vi "ReadData_9234.vi"(8 "error in":errorcluster, 11 "Module Config Selector":i16) -> (0 "error out":errorcluster, 3 "Data Array":sgl[](array[numeric]) format="%.2f")   [LabVIEW 2017, in "BOP_VibAPI_4.lvlib"]
uses:
  <vilib>/addons/InsightCM/Devices/Shared/Cms/Fpga/Acquisition/source/subVIs/VibAPI_4/BOP_VibAPI_4.lvlib
  <vilib>/rvi/eio/common/nirviEmuTemplateMethod_errors.vi
  <vilib>/eio/EIONode/EIONode.xnode
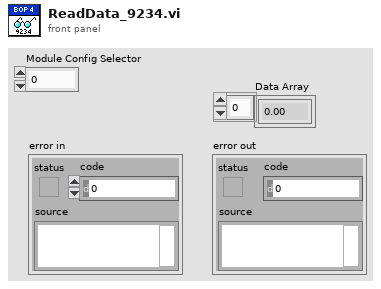
[diagram p1: front panel]
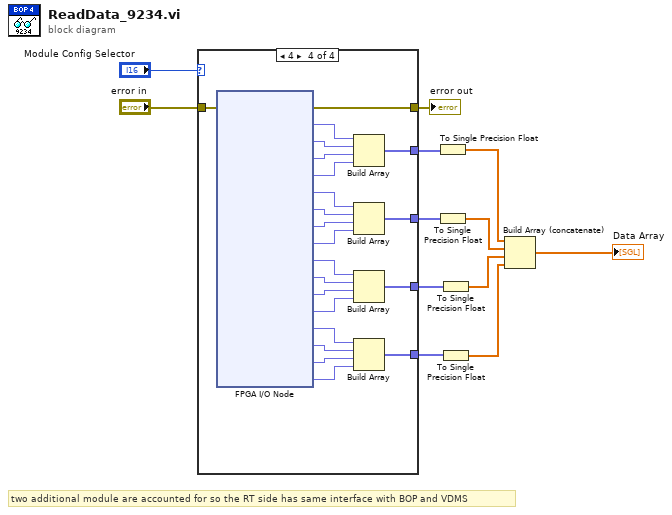
[diagram p0: block diagram]
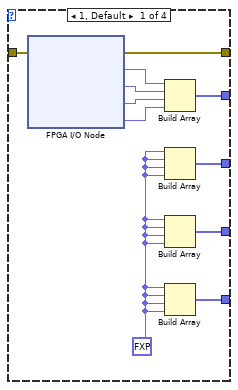
[diagram p2: hidden frame]
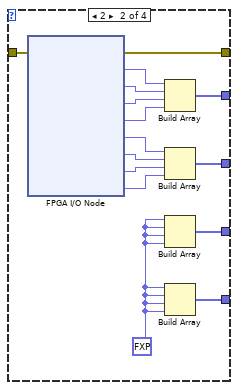
[diagram p3: hidden frame]
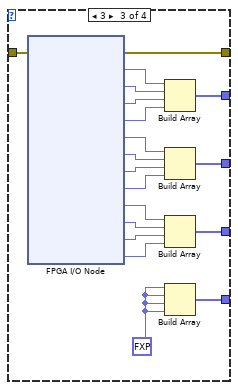
[diagram p4: hidden frame]
diagram:
  # "two additional module are accounted for so the RT side has same interface with BOP and VDMS"
  n1 = case shown="4" "Module Config Selector" {
    tunnel: "error in" -> [w20 w35 w54 w76]
    tunnel: [w19 w34 w53 w75] -> w11
    tunnel: [w18 w33 w52 w74] -> w8
    tunnel: [w17 w32 w51 w73] -> w6
    tunnel: [w16 w31 w50 w72] -> w4
    tunnel: [w15 w27 w43 w62] -> w2
    frame 1, Default {
      w13 = fxp<+/-,24,7> 0.0 ("Mod3/AI2")
      n2 = xnode "FPGA I/O Node"("error in"=w20) -> ("error out"=w19:errorcluster, "Mod1/AI0"=w21:fxp<+/-,24,4>, "Mod1/AI1"=w23:fxp<+/-,24,4>, "Mod1/AI2"=w22:fxp<+/-,24,4>, "Mod1/AI3"=w14:fxp<+/-,24,4>)  [unwired: 4 in, 4 out]
      n3 = Build Array(w21, w23, w22, w14) -> (w18:fxp<+/-,24,4>[])
      n4 = Build Array(w13, w13, w13, w13) -> (w17:fxp<+/-,24,7>[])
      n5 = Build Array(w13, w13, w13, w13) -> (w16:fxp<+/-,24,7>[])
      n6 = Build Array(w13, w13, w13, w13) -> (w15:fxp<+/-,24,7>[])
    }
    frame 2 {
      w24 = fxp<+/-,24,7> 0.0 ("Mod3/AI2")
      n7 = xnode "FPGA I/O Node"("error in"=w35) -> ("error out"=w34:errorcluster, "Mod1/AI0"=w36:fxp<+/-,24,4>, "Mod1/AI1"=w38:fxp<+/-,24,4>, "Mod1/AI2"=w37:fxp<+/-,24,4>, "Mod1/AI3"=w26:fxp<+/-,24,4>, "Mod2/AI0"=w30:fxp<+/-,24,4>, "Mod2/AI1"=w29:fxp<+/-,24,4>, "Mod2/AI2"=w28:fxp<+/-,24,4>, "Mod2/AI3"=w25:fxp<+/-,24,4>)  [unwired: 8 in, 8 out]
      n8 = Build Array(w36, w38, w37, w26) -> (w33:fxp<+/-,24,4>[])
      n9 = Build Array(w30, w29, w28, w25) -> (w32:fxp<+/-,24,4>[])
      n10 = Build Array(w24, w24, w24, w24) -> (w31:fxp<+/-,24,7>[])
      n11 = Build Array(w24, w24, w24, w24) -> (w27:fxp<+/-,24,7>[])
    }
    frame 3 {
      w39 = fxp<+/-,24,7> 0.0 ("Mod3/AI2")
      n12 = xnode "FPGA I/O Node"("error in"=w54) -> ("error out"=w53:errorcluster, "Mod1/AI0"=w55:fxp<+/-,24,4>, "Mod1/AI1"=w57:fxp<+/-,24,4>, "Mod1/AI2"=w56:fxp<+/-,24,4>, "Mod1/AI3"=w42:fxp<+/-,24,4>, "Mod2/AI0"=w49:fxp<+/-,24,4>, "Mod2/AI1"=w48:fxp<+/-,24,4>, "Mod2/AI2"=w47:fxp<+/-,24,4>, "Mod2/AI3"=w41:fxp<+/-,24,4>, "Mod3/AI0"=w46:fxp<+/-,24,4>, "Mod3/AI1"=w45:fxp<+/-,24,4>, "Mod3/AI2"=w44:fxp<+/-,24,4>, "Mod3/AI3"=w40:fxp<+/-,24,4>)  [unwired: 12 in, 12 out]
      n13 = Build Array(w55, w57, w56, w42) -> (w52:fxp<+/-,24,4>[])
      n14 = Build Array(w49, w48, w47, w41) -> (w51:fxp<+/-,24,4>[])
      n15 = Build Array(w46, w45, w44, w40) -> (w50:fxp<+/-,24,4>[])
      n16 = Build Array(w39, w39, w39, w39) -> (w43:fxp<+/-,24,7>[])
    }
    frame 4 {
      n17 = xnode "FPGA I/O Node"("error in"=w76) -> ("error out"=w75:errorcluster, "Mod1/AI0"=w77:fxp<+/-,24,4>, "Mod1/AI1"=w79:fxp<+/-,24,4>, "Mod1/AI2"=w78:fxp<+/-,24,4>, "Mod1/AI3"=w61:fxp<+/-,24,4>, "Mod2/AI0"=w71:fxp<+/-,24,4>, "Mod2/AI1"=w70:fxp<+/-,24,4>, "Mod2/AI2"=w69:fxp<+/-,24,4>, "Mod2/AI3"=w60:fxp<+/-,24,4>, "Mod3/AI0"=w68:fxp<+/-,24,4>, "Mod3/AI1"=w67:fxp<+/-,24,4>, "Mod3/AI2"=w66:fxp<+/-,24,4>, "Mod3/AI3"=w59:fxp<+/-,24,4>, "Mod4/AI0"=w65:fxp<+/-,24,4>, "Mod4/AI1"=w64:fxp<+/-,24,4>, "Mod4/AI2"=w63:fxp<+/-,24,4>, "Mod4/AI3"=w58:fxp<+/-,24,4>)  [unwired: 16 in, 16 out]
      n18 = Build Array(w77, w79, w78, w61) -> (w74:fxp<+/-,24,4>[])
      n19 = Build Array(w71, w70, w69, w60) -> (w73:fxp<+/-,24,4>[])
      n20 = Build Array(w68, w67, w66, w59) -> (w72:fxp<+/-,24,4>[])
      n21 = Build Array(w65, w64, w63, w58) -> (w62:fxp<+/-,24,4>[])
    }
  }
  "error out" <- w11
  n22 = To Single Precision Float(number=w8) -> (single precision float=w7:sgl[])
  n23 = To Single Precision Float(number=w6) -> (single precision float=w5:sgl[])
  n24 = To Single Precision Float(number=w4) -> (single precision float=w3:sgl[])
  n25 = To Single Precision Float(number=w2) -> (single precision float=w1:sgl[])
  n26 = Build Array (concatenate)(w7, w5, w3, w1) -> (→"Data Array":sgl[])
